vi "Create Auto Folder Path.vi"(1 "Parent Folder Path":path) -> (0 "Auto Folder Path":path)   [LabVIEW 2024, in "Auto Modo.lvlib"]
uses:
  Auto Modo.lvlib
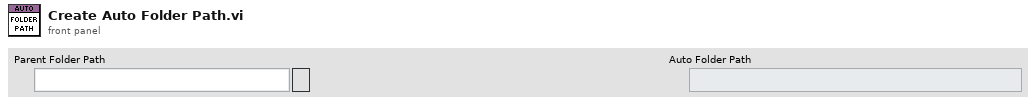
[diagram p1: front panel]
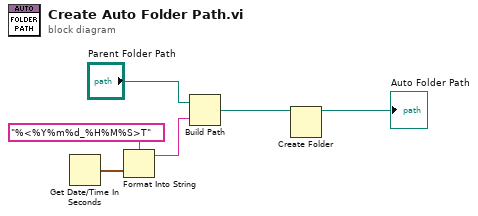
[diagram p0: block diagram]
diagram:
  n1 = Get Date/Time In Seconds() -> (seconds since 1Jan1904=w5:timestamp)
  n2 = Format Into String(format string="%<%Y%m%d_%H%M%S>T", w5) -> (resulting string=w3:string)  [unwired: 2 in, 1 out]
  n3 = Build Path(base path="Parent Folder Path", name or relative path=w3) -> (appended path=w2:path)
  n4 = Create Folder(path (use dialog)=w2) -> (created path=→"Auto Folder Path":path)  [unwired: 2 in, 2 out]
